vi "dtrig.vi"(1 "C":bool, 2 "RESET":bool, 3 "Cluster":T2) -> (0 "output cluster":T1)   [LabVIEW 2017]
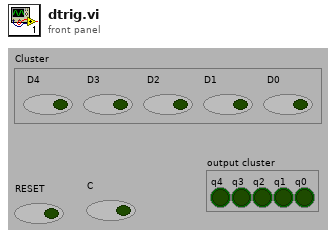
[diagram p1: front panel]
types:
  T1 = cluster{"q4":bool, "q3":bool, "q2":bool, "q1":bool, "q0":bool}
  T2 = cluster{" D4":bool, " D3":bool, " D2":bool, "D1":bool, " D0":bool}
  T3 = cluster{"q":bool, "q":bool, "q":bool, "q":bool, "q":bool}
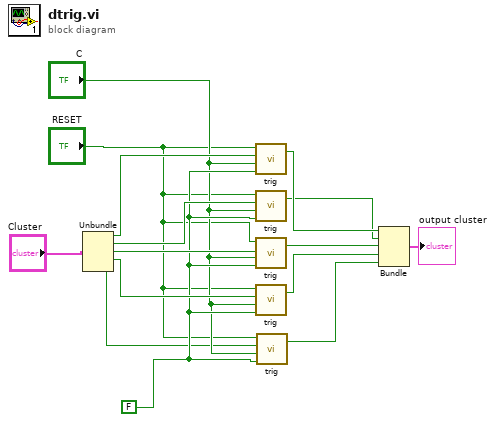
[diagram p0: block diagram]
diagram:
  w5 = FALSE
  n1 = Unbundle("Cluster") -> ("D4"=w14:bool, "D3"=w13:bool, "D2"=w12:bool, "D1"=w11:bool, "D0"=w2:bool)
  n2 = call "trig.vi"("s"=w5, "c"="C", "d"=w14, "r"="RESET") -> ("q"=w10:bool)  [unwired: 1 out]
  n3 = call "trig.vi"("s"=w5, "c"="C", "d"=w13, "r"="RESET") -> ("q"=w9:bool)  [unwired: 1 out]
  n4 = call "trig.vi"("s"=w5, "c"="C", "d"=w12, "r"="RESET") -> ("q"=w8:bool)  [unwired: 1 out]
  n5 = call "trig.vi"("s"=w5, "c"="C", "d"=w11, "r"="RESET") -> ("q"=w7:bool)  [unwired: 1 out]
  n6 = call "trig.vi"("s"=w5, "c"="C", "d"=w2, "r"="RESET") -> ("q"=w1:bool)  [unwired: 1 out]
  n7 = Bundle("q"=w10, "q"=w9, "q"=w8, "q"=w7, "q"=w1) -> (→"output cluster":T3)  [unwired: 1 out]
